vi "Clock Frequency generator hilbert without wavepond.vi"(10 "k-space signal in":u16[](array[numeric])=array[5000 elements]) -> (3 "Zero Crossing Resample Index":i32[](graph))   [LabVIEW 2014]
uses:
  <vilib>/Analysis/6fits.llb/Curve Fitting Criteria.ctl
  <vilib>/Analysis/baseanly.llb/Mean (DBL).vi
  <vilib>/measure/matone.llb/Extract Single Tone Information 1 Chan.vi
  <vilib>/measure/maresamp.llb/Resample Waveform (single shot).vi
  <vilib>/Analysis/NI_AALBase.lvlib
  <vilib>/Analysis/NI_AALPro.lvlib
  <vilib>/measure/NI_MAPro.lvlib
  <vilib>/ptbypt/NI_PtbyPt.lvlib
panel:
  in  "Sample Rate (MS/s)":dbl=180.0
  # "4385 updates is the maximum number for the clock of\nthe output card which updates every 11.4 ns"
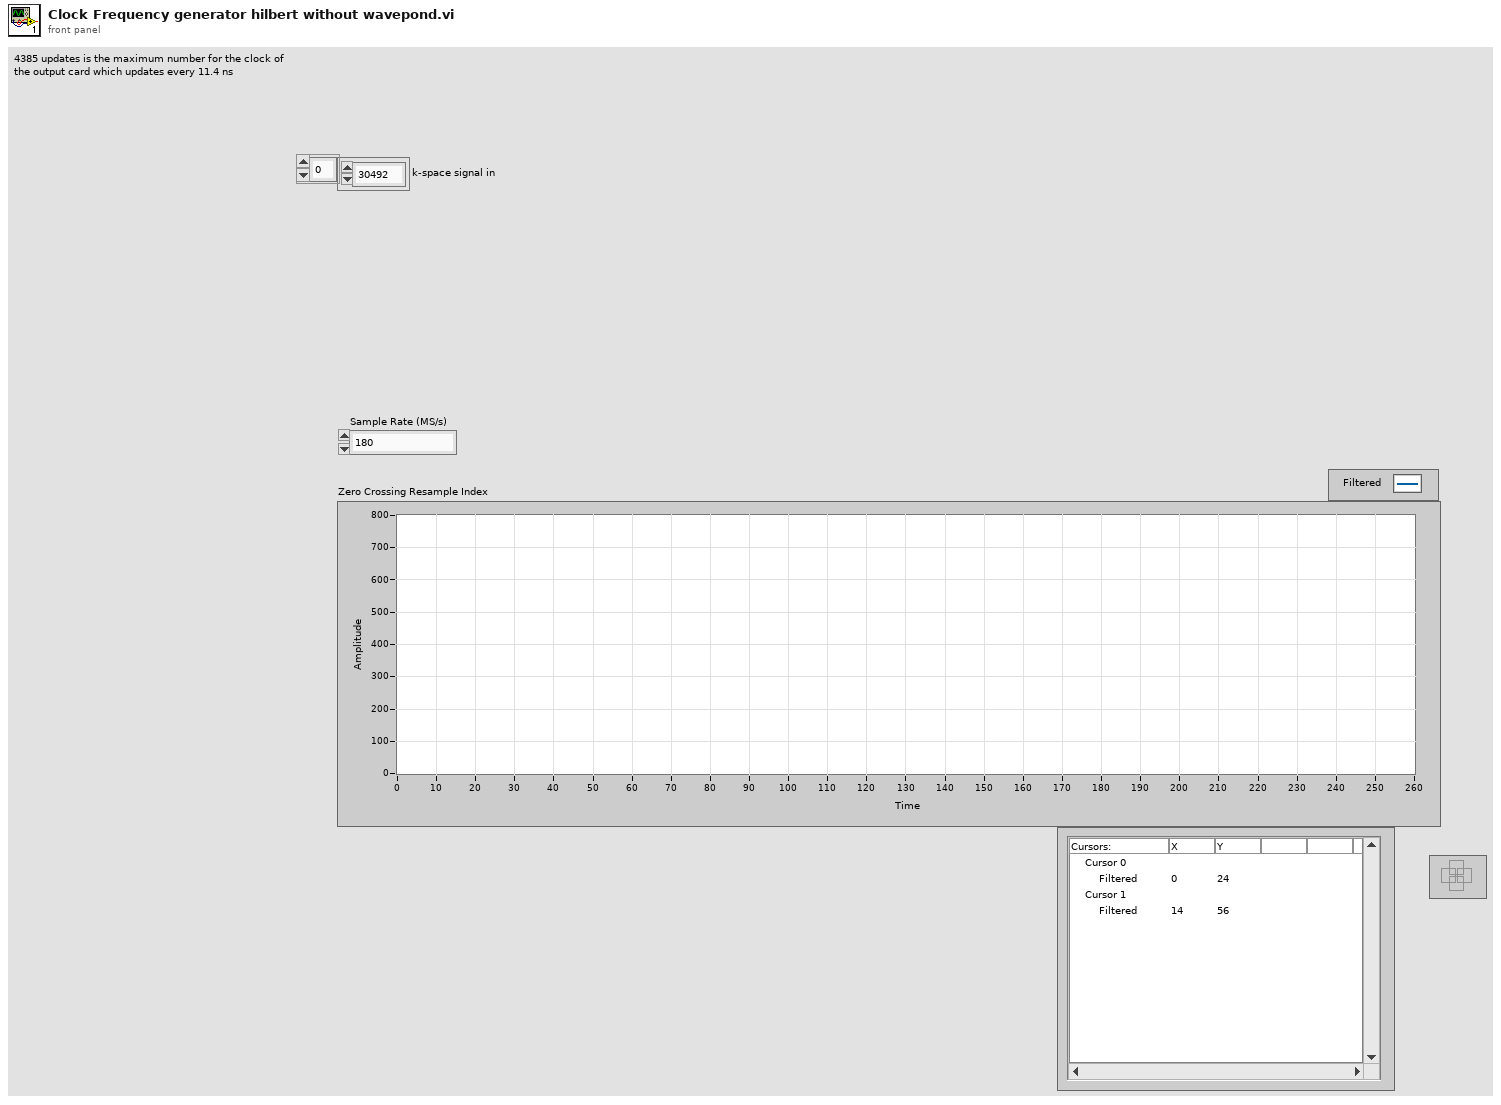
[diagram p1: front panel]
types:
  T1 = typedef "NI_AALPro.lvlib/Curve Fitting Criteria.ctl" = u16
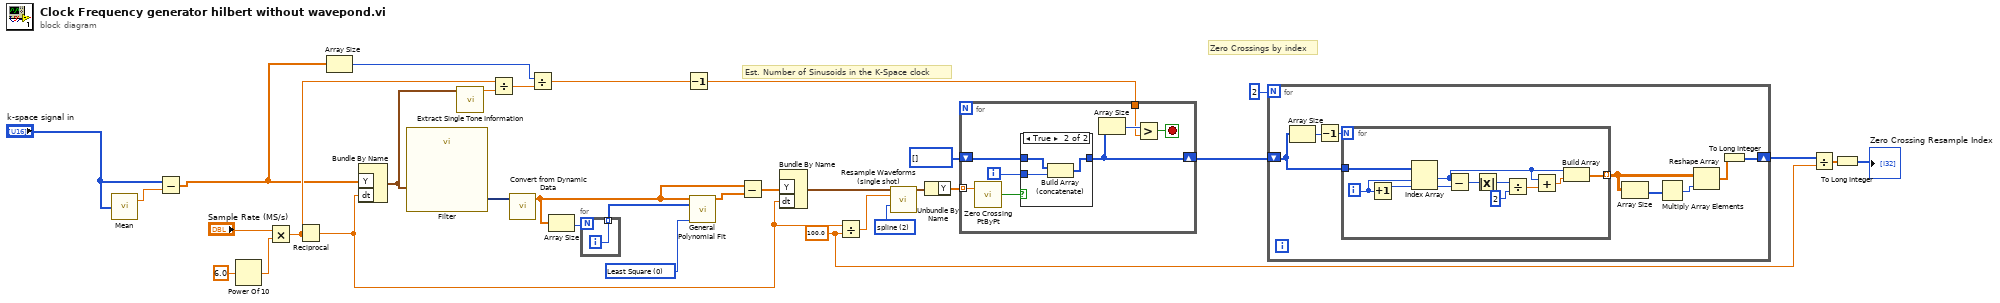
[diagram p0: block diagram]
diagram:
  w4 = 100.0 ("y")
  w21 = u16 2 items=["coerce", "linear", "spline", "FIR filter"] ("interpolation mode")
  w26 = T1 0 items=["Least Square", "Least Absolute Residual", "Bisquare"] ("method")
  # "Zero Crossings by index"
  # "Est. Number of Sinusoids in the K-Space clock"
  n1 = call-poly <vilib>:"Mean.vi"("X"="k-space signal in") -> ("mean"=w30:dbl)  [unwired: 1 out]
  n2 = Subtract(x="k-space signal in", y=w30) -> (x-y=w10:dbl[])
  n3 = Power Of 10(x=6.0) -> (10^x=w31:dbl)
  n4 = Multiply(x="Sample Rate (MS/s)", y=w31) -> (x*y=w14:dbl)
  n5 = Reciprocal(x=w14) -> (1/x=w20:dbl)
  n6 = Array Size(array=w10) -> (size(s)=w11:i32)
  n7 = Bundle By Name("Y"=w10, "dt"=w20) -> (w13:waveform(dbl))  [unwired: 1 in]
  n8 = call "Filter"("Signal"=w13) -> ("Filtered Signal"=w29:dynamicdata)  [unwired: 9 in, 1 out]
  n9 = call-poly <vilib>:"Extract Single Tone Information.vi"("time signal in"=w13) -> ("detected frequency"=w15:dbl)  [unwired: 5 in, 5 out]
  n10 = Divide(x=w14, y=w15) -> (x/y=w12:dbl)
  n11 = call "Convert from Dynamic Data"("Dynamic Data Type"=w29) -> ("Array"=w25:dbl[])  [unwired: 3 in]
  n12 = Divide(x=w11, y=w12) -> (x/y=w9:dbl)
  n13 = Array Size(array=w25) -> (size(s)=w28:i32)
  n14 = for {
    N: w28 -> [_]
    tunnel: [w34] -> w27 mode=indexing
    i -> [w34]
  }
  n15 = Decrement(x=w9) -> (x-1=w8:dbl)
  n16 = call <vilib>:"General Polynomial Fit.vi"("Y"=w25, "X"=w27, "method"=w26) -> ("Best Polynomial Fit"=w24:dbl[])  [unwired: 9 in, 3 out]
  n17 = Subtract(x=w25, y=w24) -> (x-y=w23:dbl[])
  n18 = Bundle By Name("Y"=w23, "dt"=w20) -> (w22:waveform(dbl))  [unwired: 1 in]
  n19 = Divide(x=w20, y=w4) -> (x/y=w19:dbl)
  n20 = call-poly <vilib>:"Resample Waveforms (single shot).vi"("waveform in"=w22, "dt"=w19, "interpolation mode"=w21) -> ("resampled waveform out"=w18:waveform(dbl))  [unwired: 9 in, 3 out]
  n21 = Unbundle By Name(w18) -> ("Y"=w16:dbl[])
  n22 = for {
    tunnel: w16 -> [w42] mode=indexing
    shift-right: [w38] -> w7
    shift-left: i32[] [] -> [w39]
    tunnel: w8 -> [w35]
    i -> [w40]
    stop <- w37 stop-if-true
    n23 = call <vilib>:"Zero Crossing PtByPt.vi"("input data point"=w42) -> ("crossing"=w41:bool)  [unwired: 2 in]
    n24 = case shown="True" w41 {
      tunnel: w40 -> [_ w46]
      tunnel: w39 -> [w43 w45]
      tunnel: [w43 w44] -> w38
      frame False {
      }
      frame True {
        n25 = Build Array (concatenate)(w45, w46) -> (w44:i32[])
      }
    }
    n26 = Array Size(array=w38) -> (size(s)=w36:i32)
    n27 = Greater?(x=w36, y=w35) -> (0:w37:bool)
  }
  n28 = for {
    N: 2 -> [_]
    shift-right: [w47] -> w5
    shift-left: w7 -> [w54]
    n29 = Array Size(array=w54) -> (size(s)=w53:i32)
    n30 = Decrement(x=w53) -> (x-1=w52:i32)
    n31 = for {
      N: w52 -> [_]
      tunnel: w54 -> [w64]
      tunnel: [w55] -> w51 mode=indexing
      i -> [w58]
      n32 = Increment(x=w58) -> (x+1=w65:i32)
      n33 = Index Array(array=w64, index #1=w58, index #2=w65) -> (element #1=w56:i32, element #2=w63:i32)
      n34 = Subtract(x=w56, y=w63) -> (x-y=w62:i32)
      n35 = Absolute Value(x=w62) -> (abs(x)=w61:i32)
      n36 = Divide(x=w61, y=2) -> (x/y=w59:dbl)
      n37 = Add(x=w56, y=w59) -> (x+y=w57:dbl)
      n38 = Build Array(w56, w57) -> (w55:dbl[])
    }
    n39 = Array Size(array=w51) -> (size(s)=w49:i32[])
    n40 = Multiply Array Elements(1:w49) -> (0:w50:i32)
    n41 = Reshape Array(w51, w50) -> (w48:dbl[])
    n42 = To Long Integer(number=w48) -> (32bit integer=w47:i32[])
  }
  n43 = Divide(x=w5, y=w4) -> (x/y=w3:dbl[])
  n44 = To Long Integer(number=w3) -> (32bit integer=→"Zero Crossing Resample Index":i32[])
